vi "New Off Wire Message from JSON.vi"(2 "error in":errorcluster, 3 "JSON string":string) -> (0 "error out":errorcluster, 1 "Off Wire Message":T1)   [LabVIEW 2016]
uses:
  Off Wire Message.ctl
  Generic Message.ctl
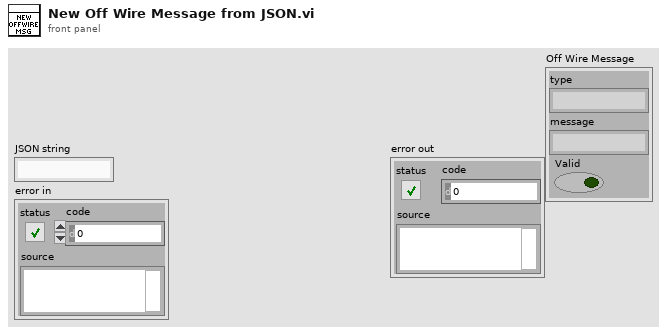
[diagram p1: front panel]
types:
  T1 = typedef "Off Wire Message.ctl" = cluster{"type":string, "message":string, "Valid":bool}
  T2 = typedef "Generic Message.ctl" = cluster{"type":string, "message":string}
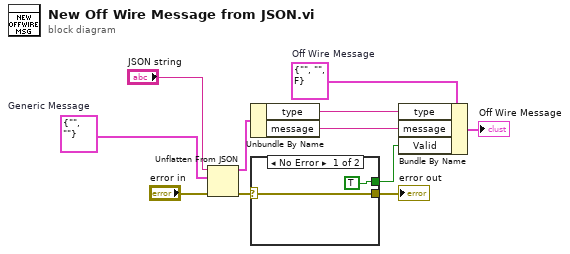
[diagram p0: block diagram]
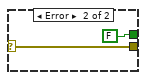
[diagram p2: hidden frame]
diagram:
  w1 = T2 {"type"="", "message"=""}  # Generic Message
  w3 = T1 {"type"="", "message"="", "Valid"=FALSE}  # Off Wire Message
  n1 = Unflatten From JSON(JSON string="JSON string", type and defaults=w1, error in (no error)="error in") -> (value=w10:T2, error out=w8:errorcluster)  [unwired: 4 in]
  n2 = Unbundle By Name(w10) -> ("type"=w6:string, "message"=w5:string)
  n3 = case shown="No Error" w8 {
    selector: w8 -> [w13 w15]
    tunnel: [w13 w15] -> w7
    tunnel: [TRUE FALSE] -> w4
    frame No Error {
    }
    frame Error {
    }
  }
  "error out" <- w7
  n4 = Bundle By Name(cluster=w3, "type"=w6, "message"=w5, "Valid"=w4) -> (→"Off Wire Message":T1)
